vi "Write QD Settings.vi"(8 "error in (no error)":errorcluster, 10 "QD Settings":T1, 11 "Dot Settings in":refnum<class "Dot Settings.lvclass">) -> (0 "error out":errorcluster, 3 "Dot Settings out":refnum<class "Dot Settings.lvclass">)   [LabVIEW 2019, in "Dot Settings.lvclass"]
uses:
  Dot Settings.lvclass
  0ad6e9e6-7c00-45cc-9d14-b1bd192a2785.vi
  TypeDefs/QD Settings.ctl
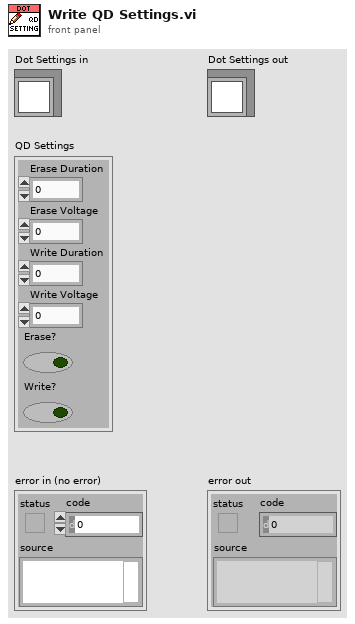
[diagram p1: front panel]
types:
  T1 = typedef "Dot Settings.lvclass/QD Settings.ctl" = cluster{"Erase Duration":dbl, "Erase Voltage":dbl, "Write Duration":dbl, "Write Voltage":dbl, "Erase?":bool, "Write?":bool}
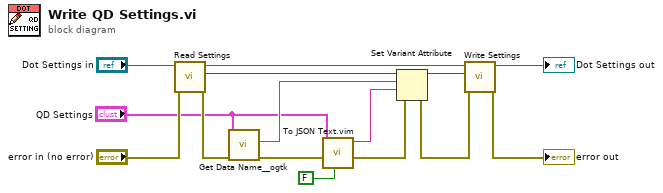
[diagram p0: block diagram]
diagram:
  n1 = call "Read Settings.vi"("error in (no error)"="error in (no error)", "Dot Settings in"="Dot Settings in") -> ("error out"=w9:errorcluster, "Settings"=w12:variant, "Dot Settings out"=w11:refnum<class "Dot Settings.lvclass">)  [unwired: 7 in]
  n2 = call <userlib>:"Get Data Name__ogtk.vi"("error in (no error)"=w9, "Data"="QD Settings") -> ("error out"=w5:errorcluster, "Data Name"=w13:string)  [unwired: 7 in, 1 out]
  n3 = call "To JSON Text.vim"("Pretty Print?"=FALSE, "error in (no error)"=w5, "Anything"="QD Settings") -> ("error out"=w4:errorcluster, "<JSON>"=w2:string)  [unwired: 7 in]
  n4 = Set Variant Attribute(Variant=w12, name=w13, value=w2, error in=w4) -> (Variant out=w10:variant, error out=w8:errorcluster)  [unwired: 1 out]
  n5 = call "Write Settings.vi"("error in (no error)"=w8, "Settings"=w10, "Dot Settings in"=w11) -> ("error out"=→"error out":errorcluster, "Dot Settings out"=→"Dot Settings out":refnum<class "Dot Settings.lvclass">)  [unwired: 7 in]
